vi "Mouse Write.vi"(3 "Write Address":u8 format="%x", 4 "Timeout (ms)":i32=100, 5 "FPGA VI Reference In":refnum<k20>) -> (0 "Timed out?":bool, 2 "FPGA VI Reference Out":refnum<k20>)   [LabVIEW 2012]
uses:
  <vilib>/Utility/error.llb/Error Cluster From Error Code.vi
  <vilib>/rvi/errors/niLvFpgaAdjustHostInterfaceError.vi
  <vilib>/rvi/interface/nirviReadWriteControl/nirviReadWriteControl.xnode
  NiFpgaLv.dll
  <vilib>/rvi/interface/Simulation/niFpgaSimulationCallBeginRW.vi
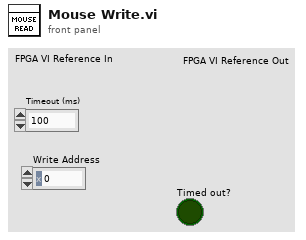
[diagram p1: front panel]
types:
  T1 = enum16{"idle", "set idle", "begin", "write", "read", "power down", "reset"}
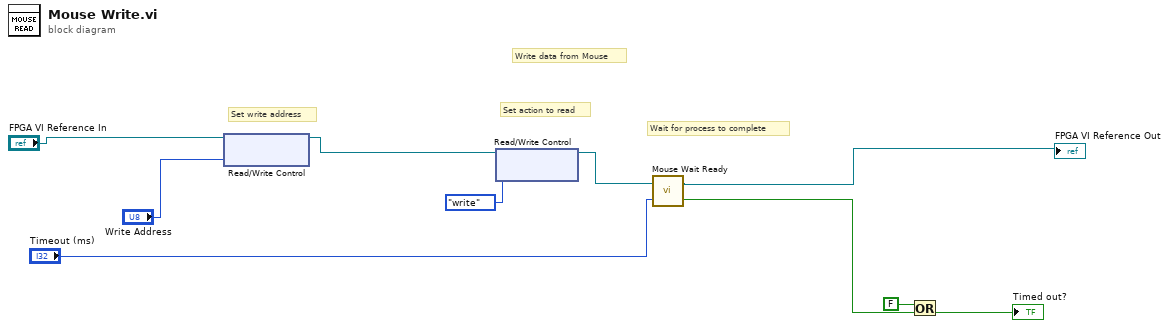
[diagram p0: block diagram]
diagram:
  # "Wait for process to complete"
  # "Set write address"
  # "Set action to read"
  # "Write data from Mouse"
  n1 = xnode "Read/Write Control"("FPGA VI Reference In"="FPGA VI Reference In", "Read Address"="Write Address") -> ("FPGA VI Reference Out"=w3:refnum<k20>)  [unwired: 1 in, 1 out]
  n2 = xnode "Read/Write Control"("FPGA VI Reference In"=w3, "Mouse Action"=T1."write") -> ("FPGA VI Reference Out"=w2:refnum<k20>)  [unwired: 1 in, 1 out]
  n3 = call "Mouse Wait Ready.vi"("Timeout (ms)"="Timeout (ms)", "Refnum in"=w2) -> ("Timeout"=w8:bool, "Refnum out"=→"FPGA VI Reference Out":refnum<k20>)
  n4 = Or(x=FALSE, y=w8) -> (x .or. y?=→"Timed out?":bool)
